vi "SetParamWavePulseRiseTime.vi"(1 "Selection":u16(ring) items=["Value", "Default", "Minimum", "Maximum"], 3 "error in (no error)":errorcluster, 4 "Rise Time [s]":dbl=1e-09 format="%#_16g", 5 "ParamWave Name":string, 6 "VISA resource name":refnum<visa-resource-name>) -> (0 "error out":errorcluster, 2 "VISA resource name out":refnum<visa-resource-name>)   [LabVIEW 2020, in "Active Technologies AWG3000.lvlib"]
uses:
  Active Technologies AWG3000.lvlib
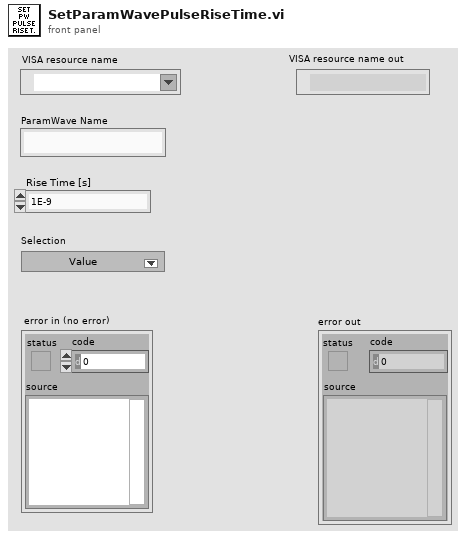
[diagram p1: front panel]
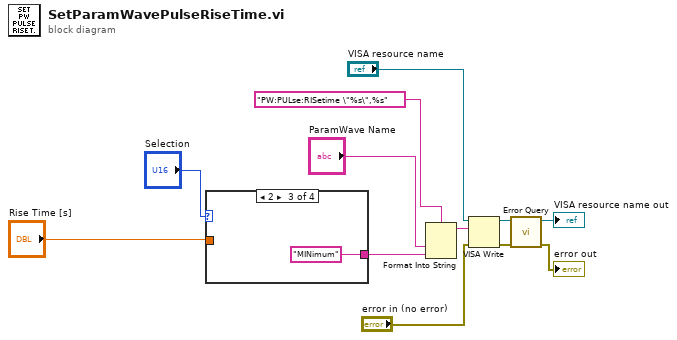
[diagram p0: block diagram]
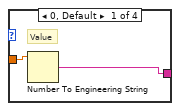
[diagram p2: hidden frame]
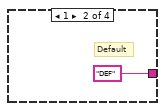
[diagram p3: hidden frame]
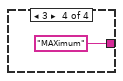
[diagram p4: hidden frame]
diagram:
  n1 = case shown="2" "Selection" {
    tunnel: [w14 "DEF" ("write buffer") "MINimum" ("write buffer") "MAXimum" ("write buffer")] -> w3
    tunnel: "Rise Time [s]" -> [w13 _ _ _]
    frame 0, Default {
      # "Value"
      n2 = Number To Engineering String(4:w13) -> (0:w14:string)  [unwired: 3 in]
    }
    frame 1 {
      # "Default"
    }
    frame 2 {
    }
    frame 3 {
    }
  }
  n3 = Format Into String(format string="PW:PULse:RISetime \"%s\",%s" ("write buffer"), "ParamWave Name", w3) -> (resulting string=w2:string)  [unwired: 2 in, 1 out]
  n4 = VISA Write(VISA resource name="VISA resource name", write buffer=w2, error in (no error)="error in (no error)") -> (VISA resource name out=w10:refnum<visa-resource-name>, error out=w9:errorcluster)  [unwired: 1 out]
  n5 = call "Error Query.vi"("error in (no error)"=w9, "VISA resource name"=w10) -> ("error out"=→"error out":errorcluster, "VISA resource name out"=→"VISA resource name out":refnum<visa-resource-name>)  [unwired: 6 in, 2 out]
